vi "Encoder Event Example.vi"() -> ()   [LabVIEW 2012, in "Phidget Encoder.lvlib"]
uses:
  <instrlib>/Phidgets/Phidget Encoder/Phidget Encoder.lvlib
  <instrlib>/Phidgets/Phidget Encoder/Public/EncoderStart.vi
  <instrlib>/Phidgets/Phidget Encoder/Public/EncoderClose.vi
  <instrlib>/Phidgets/Phidget Common/Phidget Common.lvlib
panel:
  out "Index Trigged":bool
  out "Time Change (ms)":dbl caption="Time Change" format="%.2f"
  out "Pos Change":i32
  in  "stop":bool
  out "Serial Number Return":i32
  in  "Device Info":T1={"Serial Number"=-1, "Channel"=0, "Port"=0}
  out "error out":errorcluster
  # "Be sure to use this stop button to stop the program.\nIf you use the \"Abort Execution\" button, you will\nneed to use PhidgetResetLibrary.vi or restart Labview \nin order for any Phidgets to work."
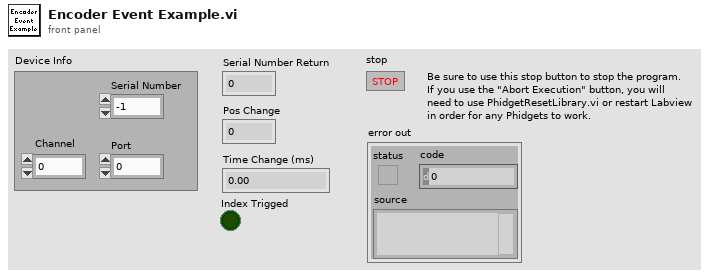
[diagram p1: front panel]
types:
  T1 = cluster{"Serial Number":i32, "Channel":i32, "Port":i32}
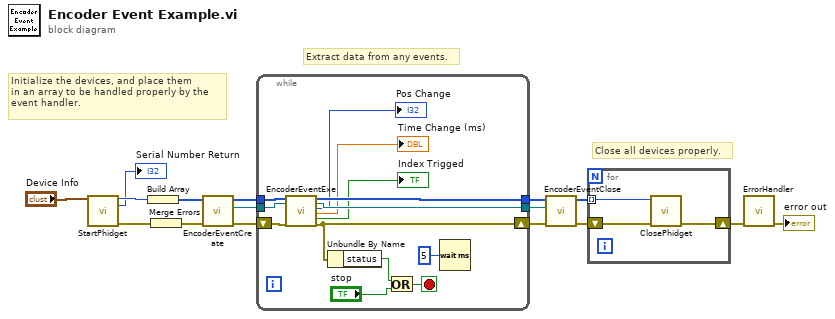
[diagram p0: block diagram]
diagram:
  # "Close all devices properly."
  # "Extract data from any events."
  # "Initialize the devices, and place them\nin an array to be handled properly by the\nevent handler."
  n1 = call-poly <instrlib>:"StartPhidget.vi"("Device Info"="Device Info") -> ("Phidget ID"=w5:u64, "Serial Number Return"=→"Serial Number Return":i32, "error out"=w1:errorcluster)  [unwired: 11 in, 1 out]
  n2 = Build Array(w5) -> (w16:u64[])
  n3 = Merge Errors(w1) -> (w7:errorcluster)
  n4 = call <instrlib>:"EncoderEventCreate.vi"("error in (no error)"=w7, "Devices In"=w16) -> ("error out"=w9:errorcluster, "Event Registration Refnum"=w14:refnum<event-registration>, "Devices Out"=w15:u64[])  [unwired: 7 in]
  n5 = while {
    tunnel: w15 -> [w29]
    tunnel: w14 -> [w25]
    tunnel: [w20] -> w11
    shift-right: [w24] -> w10
    shift-left: w9 -> [w28]
    tunnel: [w26] -> w3
    stop <- w23 stop-if-true
    n6 = call <instrlib>:"EncoderEventExe.vi"("Devices In"=w29, "Event Registration Refnum In"=w25, "error in (no error)"=w28) -> ("Devices Out"=w26:u64[], "Event Registration Refnum Out"=w20:refnum<event-registration>, "Pos Change"=→"Pos Change":i32, "Time Change"=→"Time Change (ms)":dbl, "Index Trigged"=→"Index Trigged":bool, "error out"=w24:errorcluster)  [unwired: 8 in, 3 out]
    n7 = Unbundle By Name(w24) -> ("status"=w21:bool)
    n8 = Or(x=w21, y="stop") -> (x .or. y?=w23:bool)
    n9 = Wait (ms)(milliseconds to wait=u32 5) -> ()  [unwired: 1 out]
  }
  n10 = call <instrlib>:"EncoderEventClose.vi"("error in (no error)"=w10, "Event Registration Refnum In"=w11, "Devices In"=w3) -> ("error out"=w6:errorcluster, "Devices Out"=w4:u64[])  [unwired: 7 in]
  n11 = for {
    tunnel: w4 -> [w30] mode=indexing
    shift-right: [w32] -> w13
    shift-left: w6 -> [w31]
    n12 = call-poly <instrlib>:"ClosePhidget.vi"("error in"=w31, "Device In"=w30) -> ("error out"=w32:errorcluster)  [unwired: 9 in]
  }
  n13 = call <instrlib>:"ErrorHandler.vi"("error in"=w13) -> ("error out"=→"error out":errorcluster)  [unwired: 9 in, 1 out]
